vi "Turn Crank.vi"(0 "reference in":refnum<class "Has Coin State.lvclass">, 5 "error in (no error)":errorcluster) -> (14 "reference out":refnum<class "Has Coin State.lvclass">, 19 "error out":errorcluster)   [LabVIEW 2013, in "Has Coin State.lvclass"]
uses:
  Has Coin State.lvclass
  Gum Machine_class/Gum Machine.lvclass
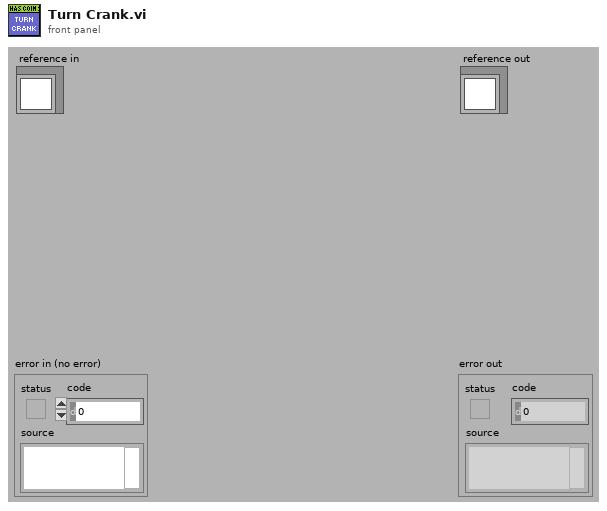
[diagram p1: front panel]
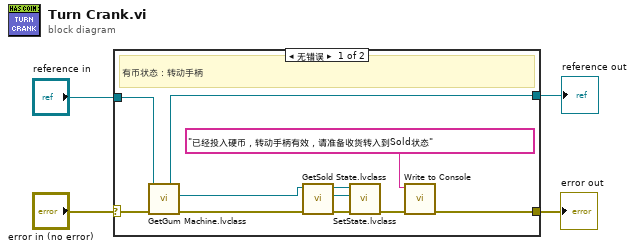
[diagram p0: block diagram]
diagram:
  n1 = case shown="无错误" "error in (no error)" {
    selector: "error in (no error)" -> [w12 w17]
    tunnel: [w15 w17] -> w3
    tunnel: [w5 w16] -> w1
    tunnel: "reference in" -> [w13 w16]
    frame No Error {
      # "有币状态：转动手柄"
      n2 = call-dynamic "GetGum Machine.lvclass.vi"("error in (no error)"=w12, "reference in"=w13) -> ("error out"=w7:errorcluster, "Gum Machine.lvclass"=w11:refnum<class "Gum Machine.lvclass">, "reference out"=w5:refnum<class "Has Coin State.lvclass">)  [unwired: 7 in]
      n3 = call-dynamic "GetSold State.lvclass.vi"("error in (no error)"=w7, "reference in"=w11) -> ("error out"=w8:errorcluster, "Sold State.lvclass"=w9:refnum<class "Sold State.lvclass">, "reference out"=w10:refnum<class "Gum Machine.lvclass">)  [unwired: 7 in]
      n4 = call-dynamic "SetState.lvclass.vi"("error in (no error)"=w8, "State.lvclass"=w9, "reference in"=w10) -> ("error out"=w6:errorcluster)  [unwired: 7 in, 1 out]
      n5 = call "Write to Console.vi"("error in (no error)"=w6, "Input"="已经投入硬币，转动手柄有效，请准备收货转入到Sold状态") -> ("error out"=w15:errorcluster)  [unwired: 9 in]
    }
    frame Error {
    }
  }
  "error out" <- w3
  "reference out" <- w1
